vi "HCC Read Write Display.vi"(7 "Read Write Control":enum16{"Read", "Write"}(ring), 8 "error in (no error)":errorcluster, 10 "Washer Input":T1={"Appliance Details"={"FileVersionInfo"={"FileVersion"="", "ProductName"="", "InternalName"="", "CompanyName"="", "LegalCopyright"="", "FileDescription"=""}, "Dishwasher Info"={"Open Cup Weight (gm):"=0.0, "Auto Cup Weight (gm):"=0.0, "Detergent-Dish:"="", "Inlet Temperature-Dish:"="", "Cycle Mode-Dish:"="", "Unit Control-Dish:"="", "Manufacturer-Dish:"=""}, "Washer Info"={"Hot Water Temperature (Fahrenheit):"="", "Cold Water Temperature (Fahrenheit):"="", "Capacity (cu.ft):"=0.0, "Initial Cloth Weight:"=0.0, "Cloth Lot:"=0, "Model Family:"="", "Program Name:"="", "Cycle Selection:"="", "Wash Temperature:"="", "Rinse Temperature:"="", "Load Size:"=""}, "File Name Output Array"=[], "Calibration Output Array"=[], "Appliance Common"={"Engineer:"="", "Model Number:"="", "Serial Number:"="", "Comments:"="", "Station ID:"="", "Technician:"="", "TR Number:"="", "Lab ID:"="", "Voltage:"="", "Water Pressure (PSI):"="", "Test Date:"="", "Computer Name:"="", "IP Address:"="", "Ambient RH:"="", "Frequency:"="", "Build:"="", "Filename:"="", "Test Type:"="", "Load Run #:"=0, "Ambient Temperature (F):"="", "File Path:"=path "", "Cycles Per Year"=60}, "Water Heater"={"Heating Mode:"=""}, "Dryer"={"Heat Setting:"="", "Washer Water Temperature (60 ± 5°F):"=60, "Water Hardness (PPM):"=17, "Dryness Setting:"="", "Dryer Type:"="", "Exhaust:"="", "Drying Cycle:"="", "Load Type:"="", "Nominal Load Weight"="", "Dryer Initial IMC Data"={"Measured IMC (lbs)"=7.0, "Actual Initial RMC (%)"=7.0, "RMC (Desired %)"=100.0, "Bone Dry Wt(lbs)"=7.0, "Tolerance(%)"=5.0, "Actual Final RMC (%)"=0.0, "CEF (lbf/kWh)"=0.0, "Minimum Weight (lbf)"=0.0, "Average Weight (lbf)"=0.0, "Maximum Weight (lbf)"=0.0, "Measured IMC In Range?"=FALSE, "Moisture Reduction Factor"=55.5, "Field Use Factor"=1.04, "Empty Dryer Cold Weigth"=0.0, "Energy Standard"=enum."D2-Automatic Dryer", "Weight Cloth (lbs)"=0.0, "Relative Moisture Content (%)"=0.0, "Relative Moisture Content - Avg (%)"=0.0}}}, "Display Data (RLT)"={"Status Color"=0, "Serial Number Display"="", "Cycle Count Display"=0, "Station Label Display"="", "Current Run Start Time Display"=0.0, "Board ID Display"="", "RPM Display"=0, "Current Display"=0.0, "Current Path Display"=path "", "Saving Display"=FALSE, "Unit Type Display"=enum."", "Total Time On Display"=0.0, "UI Button"=FALSE}} {"Display Data (RLT)"."Current Display" format="%.2f"; "Display Data (RLT)"."Cycle Count Display" format="%04d"; "Appliance Details"."Dryer"."Dryer Initial IMC Data"."Maximum Weight (lbf)" format="%03_6g"; "Appliance Details"."Dryer"."Dryer Initial IMC Data"."Average Weight (lbf)" format="%03_6g"; "Appliance Details"."Dryer"."Dryer Initial IMC Data"."Minimum Weight (lbf)" format="%03_6g"; "Appliance Details"."Dryer"."Dryer Initial IMC Data"."CEF (lbf/kWh)" format="%03_6g"; "Appliance Details"."Dryer"."Dryer Initial IMC Data"."Actual Final RMC (%)" format="%03_6g"; "Appliance Details"."Dryer"."Dryer Initial IMC Data"."Tolerance(%)" format="%0#_6g"; "Appliance Details"."Dryer"."Dryer Initial IMC Data"."Bone Dry Wt(lbs)" format="%03_6g"; "Appliance Details"."Dryer"."Dryer Initial IMC Data"."RMC (Desired %)" format="%0#_6g"; "Appliance Details"."Dryer"."Dryer Initial IMC Data"."Actual Initial RMC (%)" format="%03_6g"; "Appliance Details"."Dryer"."Dryer Initial IMC Data"."Measured IMC (lbs)" format="%0#_6g"}, 11 "File Locations In":T10) -> (0 "error out":errorcluster, 2 "Washer Output":T1={"Appliance Details"={"FileVersionInfo"={"FileVersion"="", "ProductName"="", "InternalName"="", "CompanyName"="", "LegalCopyright"="", "FileDescription"=""}, "Dishwasher Info"={"Open Cup Weight (gm):"=0.0, "Auto Cup Weight (gm):"=0.0, "Detergent-Dish:"="", "Inlet Temperature-Dish:"="", "Cycle Mode-Dish:"="", "Unit Control-Dish:"="", "Manufacturer-Dish:"=""}, "Washer Info"={"Hot Water Temperature (Fahrenheit):"="", "Cold Water Temperature (Fahrenheit):"="", "Capacity (cu.ft):"=0.0, "Initial Cloth Weight:"=0.0, "Cloth Lot:"=0, "Model Family:"="", "Program Name:"="", "Cycle Selection:"="", "Wash Temperature:"="", "Rinse Temperature:"="", "Load Size:"=""}, "File Name Output Array"=[], "Calibration Output Array"=[], "Appliance Common"={"Engineer:"="", "Model Number:"="", "Serial Number:"="", "Comments:"="", "Station ID:"="", "Technician:"="", "TR Number:"="", "Lab ID:"="", "Voltage:"="", "Water Pressure (PSI):"="", "Test Date:"="", "Computer Name:"="", "IP Address:"="", "Ambient RH:"="", "Frequency:"="", "Build:"="", "Filename:"="", "Test Type:"="", "Load Run #:"=0, "Ambient Temperature (F):"="", "File Path:"=path "", "Cycles Per Year"=60}, "Water Heater"={"Heating Mode:"=""}, "Dryer"={"Heat Setting:"="", "Washer Water Temperature (60 ± 5°F):"=60, "Water Hardness (PPM):"=17, "Dryness Setting:"="", "Dryer Type:"="", "Exhaust:"="", "Drying Cycle:"="", "Load Type:"="", "Nominal Load Weight"="", "Dryer Initial IMC Data"={"Measured IMC (lbs)"=7.0, "Actual Initial RMC (%)"=7.0, "RMC (Desired %)"=100.0, "Bone Dry Wt(lbs)"=7.0, "Tolerance(%)"=5.0, "Actual Final RMC (%)"=0.0, "CEF (lbf/kWh)"=0.0, "Minimum Weight (lbf)"=0.0, "Average Weight (lbf)"=0.0, "Maximum Weight (lbf)"=0.0, "Measured IMC In Range?"=FALSE, "Moisture Reduction Factor"=55.5, "Field Use Factor"=1.04, "Empty Dryer Cold Weigth"=0.0, "Energy Standard"=enum."D2-Automatic Dryer", "Weight Cloth (lbs)"=0.0, "Relative Moisture Content (%)"=0.0, "Relative Moisture Content - Avg (%)"=0.0}}}, "Display Data (RLT)"={"Status Color"=0, "Serial Number Display"="", "Cycle Count Display"=0, "Station Label Display"="", "Current Run Start Time Display"=0.0, "Board ID Display"="", "RPM Display"=0, "Current Display"=0.0, "Current Path Display"=path "", "Saving Display"=FALSE, "Unit Type Display"=enum."", "Total Time On Display"=0.0, "UI Button"=FALSE}} {"Display Data (RLT)"."Current Display" format="%.2f"; "Display Data (RLT)"."Cycle Count Display" format="%04d"; "Appliance Details"."Dryer"."Dryer Initial IMC Data"."Maximum Weight (lbf)" format="%03_6g"; "Appliance Details"."Dryer"."Dryer Initial IMC Data"."Average Weight (lbf)" format="%03_6g"; "Appliance Details"."Dryer"."Dryer Initial IMC Data"."Minimum Weight (lbf)" format="%03_6g"; "Appliance Details"."Dryer"."Dryer Initial IMC Data"."CEF (lbf/kWh)" format="%03_6g"; "Appliance Details"."Dryer"."Dryer Initial IMC Data"."Actual Final RMC (%)" format="%03_6g"; "Appliance Details"."Dryer"."Dryer Initial IMC Data"."Tolerance(%)" format="%0#_6g"; "Appliance Details"."Dryer"."Dryer Initial IMC Data"."Bone Dry Wt(lbs)" format="%03_6g"; "Appliance Details"."Dryer"."Dryer Initial IMC Data"."RMC (Desired %)" format="%0#_6g"; "Appliance Details"."Dryer"."Dryer Initial IMC Data"."Actual Initial RMC (%)" format="%03_6g"; "Appliance Details"."Dryer"."Dryer Initial IMC Data"."Measured IMC (lbs)" format="%0#_6g"})   [LabVIEW 2019]
uses:
  Utility/Save File/Public/Type Definitions/Save File Washer.ctl
  Utility/Save File/File Setup (Public)/Type Definition/Save File DISH Dishwasher Details.ctl
  <vilib>/Platform/fileVersionInfo.llb/FileVersionInformation.ctl
  Washer DOE/Type Definitions/DOE Appliance Common.ctl
  Utility/Custom Pallet Controls/Custom Pallet String.ctl
  Utility/Save File/File Setup (Public)/Type Definition/DPT IMC Data.ctl
  Washer DOE/Type Definitions/DOE Dryer Standard.ctl
  Utility/Save File/Public/Type Definitions/Save File Appliance Display.ctl
  Utility/Save File/Public/Type Definitions/Save File Unit Type.ctl
  Utility/Save File/File Setup (Public)/Type Definition/Save File DOE File Path Control.ctl
  Utility/Save File/File Setup (Public)/Type Definition/Save File DOE Data Save Filepaths.ctl
  Utility/Save File/Global/Save File Globals HCC.vi
  <vilib>/Utility/file.llb/Read Delimited Spreadsheet (string).vi
  <vilib>/Utility/file.llb/Write Delimited Spreadsheet (string).vi
  Utility/Save File/Save File.lvlib
  Utility/Save File/File Setup.lvlib
panel:
  out "Washer Output Debug":T1={"Appliance Details"={"FileVersionInfo"={"FileVersion"="", "ProductName"="", "InternalName"="", "CompanyName"="", "LegalCopyright"="", "FileDescription"=""}, "Dishwasher Info"={"Open Cup Weight (gm):"=0.0, "Auto Cup Weight (gm):"=0.0, "Detergent-Dish:"="", "Inlet Temperature-Dish:"="", "Cycle Mode-Dish:"="", "Unit Control-Dish:"="", "Manufacturer-Dish:"=""}, "Washer Info"={"Hot Water Temperature (Fahrenheit):"="", "Cold Water Temperature (Fahrenheit):"="", "Capacity (cu.ft):"=0.0, "Initial Cloth Weight:"=0.0, "Cloth Lot:"=0, "Model Family:"="", "Program Name:"="", "Cycle Selection:"="", "Wash Temperature:"="", "Rinse Temperature:"="", "Load Size:"=""}, "File Name Output Array"=[], "Calibration Output Array"=[], "Appliance Common"={"Engineer:"="", "Model Number:"="", "Serial Number:"="", "Comments:"="", "Station ID:"="", "Technician:"="", "TR Number:"="", "Lab ID:"="", "Voltage:"="", "Water Pressure (PSI):"="", "Test Date:"="", "Computer Name:"="", "IP Address:"="", "Ambient RH:"="", "Frequency:"="", "Build:"="", "Filename:"="", "Test Type:"="", "Load Run #:"=0, "Ambient Temperature (F):"="", "File Path:"=path "", "Cycles Per Year"=60}, "Water Heater"={"Heating Mode:"=""}, "Dryer"={"Heat Setting:"="", "Washer Water Temperature (60 ± 5°F):"=60, "Water Hardness (PPM):"=17, "Dryness Setting:"="", "Dryer Type:"="", "Exhaust:"="", "Drying Cycle:"="", "Load Type:"="", "Nominal Load Weight"="", "Dryer Initial IMC Data"={"Measured IMC (lbs)"=7.0, "Actual Initial RMC (%)"=7.0, "RMC (Desired %)"=100.0, "Bone Dry Wt(lbs)"=7.0, "Tolerance(%)"=5.0, "Actual Final RMC (%)"=0.0, "CEF (lbf/kWh)"=0.0, "Minimum Weight (lbf)"=0.0, "Average Weight (lbf)"=0.0, "Maximum Weight (lbf)"=0.0, "Measured IMC In Range?"=FALSE, "Moisture Reduction Factor"=55.5, "Field Use Factor"=1.04, "Empty Dryer Cold Weigth"=0.0, "Energy Standard"=enum."D2-Automatic Dryer", "Weight Cloth (lbs)"=0.0, "Relative Moisture Content (%)"=0.0, "Relative Moisture Content - Avg (%)"=0.0}}}, "Display Data (RLT)"={"Status Color"=0, "Serial Number Display"="", "Cycle Count Display"=0, "Station Label Display"="", "Current Run Start Time Display"=0.0, "Board ID Display"="", "RPM Display"=0, "Current Display"=0.0, "Current Path Display"=path "", "Saving Display"=FALSE, "Unit Type Display"=enum."", "Total Time On Display"=0.0, "UI Button"=FALSE}} {"Display Data (RLT)"."Current Display" format="%.2f"; "Display Data (RLT)"."Cycle Count Display" format="%04d"; "Appliance Details"."Dryer"."Dryer Initial IMC Data"."Maximum Weight (lbf)" format="%03_6g"; "Appliance Details"."Dryer"."Dryer Initial IMC Data"."Average Weight (lbf)" format="%03_6g"; "Appliance Details"."Dryer"."Dryer Initial IMC Data"."Minimum Weight (lbf)" format="%03_6g"; "Appliance Details"."Dryer"."Dryer Initial IMC Data"."CEF (lbf/kWh)" format="%03_6g"; "Appliance Details"."Dryer"."Dryer Initial IMC Data"."Actual Final RMC (%)" format="%03_6g"; "Appliance Details"."Dryer"."Dryer Initial IMC Data"."Tolerance(%)" format="%0#_6g"; "Appliance Details"."Dryer"."Dryer Initial IMC Data"."Bone Dry Wt(lbs)" format="%03_6g"; "Appliance Details"."Dryer"."Dryer Initial IMC Data"."RMC (Desired %)" format="%0#_6g"; "Appliance Details"."Dryer"."Dryer Initial IMC Data"."Actual Initial RMC (%)" format="%03_6g"; "Appliance Details"."Dryer"."Dryer Initial IMC Data"."Measured IMC (lbs)" format="%0#_6g"}
  in  "Current Display (Debug)":dbl=12.1 format="%#_13g"
  in  "Cycle Count (Debug)":i32=5
  in  "Debug":bool
  in  "Tab Control":enum32{"Page 1", "Page 2"}(tab)
  out "all rows":string[][](array[string])
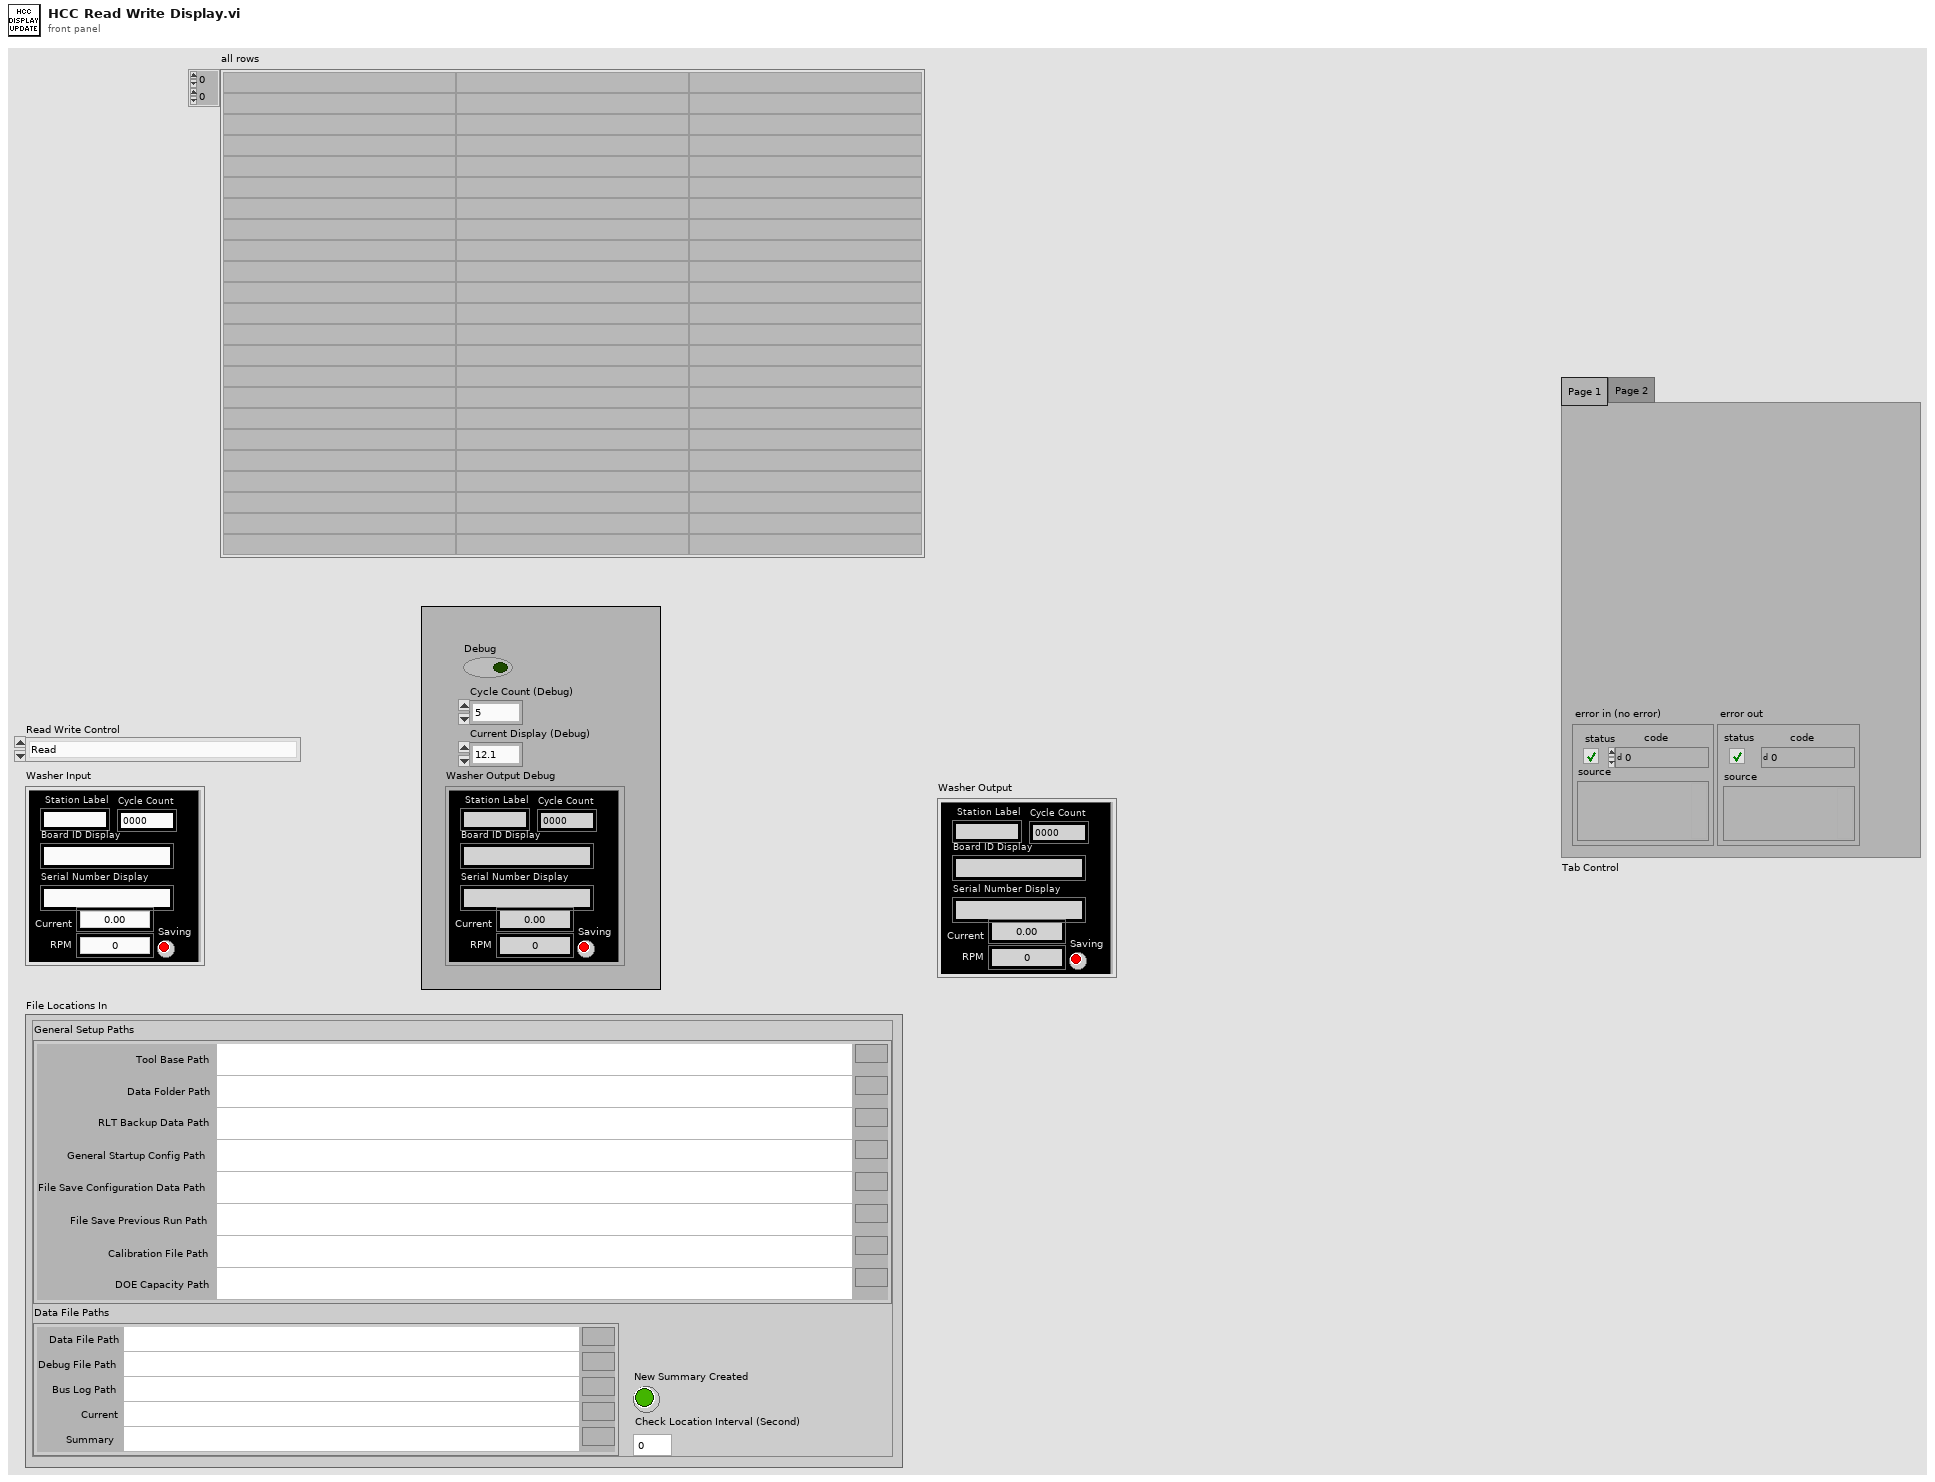
[diagram p1: front panel]
types:
  T1 = typedef "Save File.lvlib/Save File Washer.ctl" = cluster{"Appliance Details":T2, "Display Data (RLT)":T8}
  T2 = typedef "File Setup.lvlib/Save File DISH Dishwasher Details.ctl" = cluster{"FileVersionInfo":T3, "Dishwasher Info":cluster{"Open Cup Weight (gm):":dbl, "Auto Cup Weight (gm):":dbl, "Detergent-Dish:":string, "Inlet Temperature-Dish:":string, "Cycle Mode-Dish:":string, "Unit Control-Dish:":string, "Manufacturer-Dish:":string}, "Washer Info":cluster{"Hot Water Temperature (Fahrenheit):":string, "Cold Water Temperature (Fahrenheit):":string, "Capacity (cu.ft):":dbl, "Initial Cloth Weight:":dbl, "Cloth Lot:":i32, "Model Family:":string, "Program Name:":string, "Cycle Selection:":string, "Wash Temperature:":string, "Rinse Temperature:":string, "Load Size:":string}, "File Name Output Array":string[][], "Calibration Output Array":string[][], "Appliance Common":T4, "Water Heater":cluster{"Heating Mode:":string}, "Dryer":cluster{"Heat Setting:":T5, "Washer Water Temperature (60 ± 5°F):":u16, "Water Hardness (PPM):":u16, "Dryness Setting:":T5, "Dryer Type:":string, "Exhaust:":string, "Drying Cycle:":string, "Load Type:":string, "Nominal Load Weight":string, "Dryer Initial IMC Data":T6}}
  T3 = typedef "FileVersionInformation.ctl" = cluster{"FileVersion":string, "ProductName":string, "InternalName":string, "CompanyName":string, "LegalCopyright":string, "FileDescription":string}
  T4 = typedef "DOE Appliance Common.ctl" = cluster{"Engineer:":string, "Model Number:":string, "Serial Number:":string, "Comments:":string, "Station ID:":string, "Technician:":string, "TR Number:":string, "Lab ID:":string, "Voltage:":string, "Water Pressure (PSI):":string, "Test Date:":string, "Computer Name:":string, "IP Address:":string, "Ambient RH:":string, "Frequency:":string, "Build:":string, "Filename:":string, "Test Type:":string, "Load Run #:":i32, "Ambient Temperature (F):":string, "File Path:":path, "Cycles Per Year":u32}
  T5 = typedef "Custom Pallet String.ctl" = string
  T6 = typedef "DPT IMC Data.ctl" = cluster{"Measured IMC (lbs)":dbl, "Actual Initial RMC (%)":dbl, "RMC (Desired %)":dbl, "Bone Dry Wt(lbs)":dbl, "Tolerance(%)":dbl, "Actual Final RMC (%)":dbl, "CEF (lbf/kWh)":dbl, "Minimum Weight (lbf)":dbl, "Average Weight (lbf)":dbl, "Maximum Weight (lbf)":dbl, "Measured IMC In Range?":bool, "Moisture Reduction Factor":dbl, "Field Use Factor":dbl, "Empty Dryer Cold Weigth":dbl, "Energy Standard":T7, "Weight Cloth (lbs)":dbl, "Relative Moisture Content (%)":dbl, "Relative Moisture Content - Avg (%)":dbl}
  T7 = typedef "DOE Dryer Standard.ctl" = enum16{"D2-Automatic Dryer", "D2-Timer Dryer", "D1-Automatic Dryer", "D1-Timer Dryer", "Other"}
  T8 = typedef "Save File Appliance Display.ctl" = cluster{"Status Color":u32, "Serial Number Display":string, "Cycle Count Display":i32, "Station Label Display":string, "Current Run Start Time Display":dbl, "Board ID Display":string, "RPM Display":u32, "Current Display":dbl, "Current Path Display":path, "Saving Display":bool, "Unit Type Display":T9, "Total Time On Display":dbl, "UI Button":bool}
  T9 = typedef "Save File.lvlib/Save File Unit Type.ctl" = enum32{"", "Viper", "Hawk", "2015"}
  T10 = typedef "File Setup.lvlib/Save File DOE File Path Control.ctl" = cluster{"General Setup Paths":cluster{"Calibration File Path":path, "DOE Capacity Path":path, "Data Folder Path":path, "RLT Backup Data Path":path, "Tool Base Path":path, "General Startup Config Path":path, "File Save Previous Run Path":path, "File Save Configuration Data Path":path}, "Data File Paths":T11, "New Summary Created":bool, "Check Location Interval (Second)":i32}
  T11 = typedef "File Setup.lvlib/Save File DOE Data Save Filepaths.ctl" = cluster{"Data File Path":path, "Debug File Path":path, "Bus Log Path":path, "Current":path, "Summary":path}
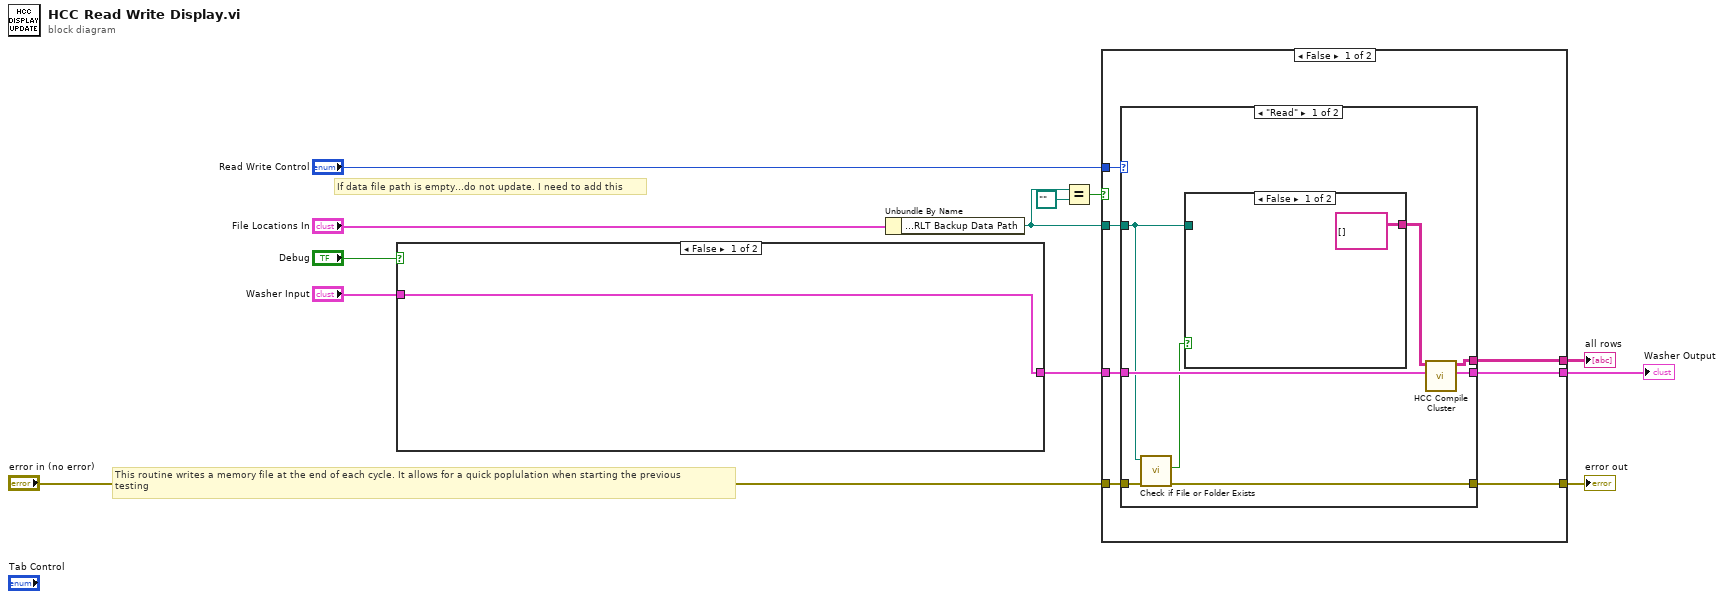
[diagram p0: block diagram]
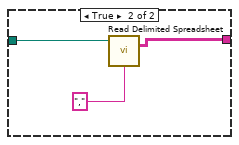
[diagram p2: hidden frame]
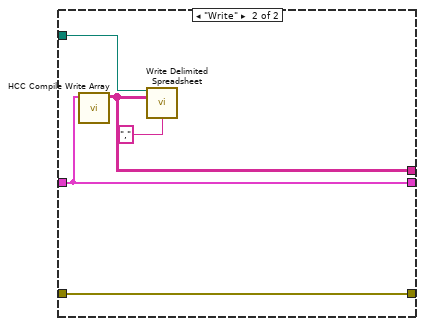
[diagram p3: hidden frame]
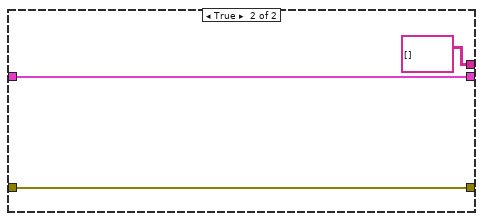
[diagram p4: hidden frame]
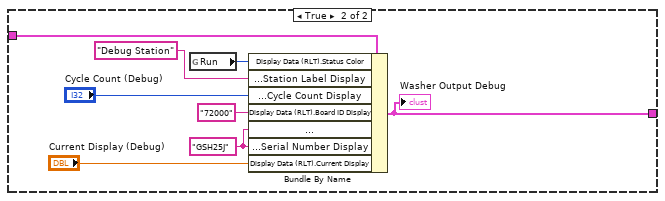
[diagram p5: hidden frame]
diagram:
  # "If data file path is empty...do not update. I need to add this"
  # "This routine writes a memory file at the end of each cycle. It allows for a quick poplulation when starting the previous \ntesting"
  n1 = case shown="False" "Debug" {
    tunnel: "Washer Input" -> [w13 w21]
    tunnel: [w13 w15] -> w6
    frame False {
    }
    frame True {
      w14 = "GSH25J" ("Serial Number Display")
      n2 = global read "Save File Globals HCC.vi" "Run"() -> (w20:u32)
      n3 = Bundle By Name(cluster=w21, "Display Data (RLT).Status Color"=w20, "Display Data (RLT).Station Label Display"="Debug Station" ("Station Label Display"), "Display Data (RLT).Cycle Count Display"="Cycle Count (Debug)", "Display Data (RLT).Board ID Display"="72000" ("Board ID Display"), "Appliance Details.Appliance Common.Serial Number:"=w14, "Display Data (RLT).Serial Number Display"=w14, "Display Data (RLT).Current Display"="Current Display (Debug)") -> (w15:T1)
      "Washer Output Debug" <- w15
    }
  }
  n4 = Unbundle By Name("File Locations In") -> ("General Setup Paths.RLT Backup Data Path"=w3:path)
  n5 = Equal?(x=w3, y=path "") -> (x = y?=w1:bool)
  n6 = case shown="False" w1 {
    tunnel: [w28 w46] -> w11
    tunnel: "Read Write Control" -> [w27 _]
    tunnel: [w26 string[][] [] ("Full Data Save")] -> w9
    tunnel: [w25 w48] -> w8
    tunnel: w6 -> [w24 w48]
    tunnel: "error in (no error)" -> [w23 w46]
    tunnel: w3 -> [w22 _]
    frame False {
      n7 = case shown="\"Read\"" w27 {
        tunnel: w22 -> [w32 w44]
        tunnel: w24 -> [w34 w43]
        tunnel: [w36 w43] -> w25
        tunnel: [w33 w41] -> w26
        tunnel: w23 -> [w31 w42]
        tunnel: [w30 w42] -> w28
        frame "Read" {
          n8 = call <vilib>:"Check if File or Folder Exists.vi"("error in (no error)"=w31, "path"=w32) -> ("error out"=w30:errorcluster, "file or folder exists?"=w29:bool)  [unwired: 7 in, 1 out]
          n9 = case shown="False" w29 {
            tunnel: [string[][] [] ("all rows") w38] -> w35
            tunnel: w32 -> [_ w39]
            frame False {
            }
            frame True {
              n10 = call-poly <vilib>:"Read Delimited Spreadsheet.vi"("file path (dialog if empty)"=w39, "delimiter (\\t)"="," ("delimiter (\\t)")) -> ("all rows"=w38:string[][])  [unwired: 8 in, 5 out]
            }
          }
          n11 = call "HCC Compile Cluster.vi"("Washer Input in"=w34, "all rows in"=w35) -> ("Washer Input out"=w36:T1, "all rows out"=w33:string[][])  [unwired: 8 in]
        }
        frame "Write" {
          n12 = call "HCC Compile Write Array.vi"("Washer Input"=w43) -> ("Full Data Save"=w41:string[][])  [unwired: 10 in]
          n13 = call-poly <vilib>:"Write Delimited Spreadsheet.vi"("file path (dialog if empty)"=w44, "2D data"=w41, "delimiter (\\t)"="," ("delimiter (\\t)")) -> ()  [unwired: 11 in, 2 out]
        }
      }
    }
    frame True {
    }
  }
  "error out" <- w11
  "Washer Output" <- w8
  "all rows" <- w9
